vi "location calculator.vi"() -> ()   [LabVIEW 2015]
panel:
  out "1-D Array of Real":dbl[](array[numeric])
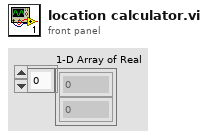
[diagram p1: front panel]
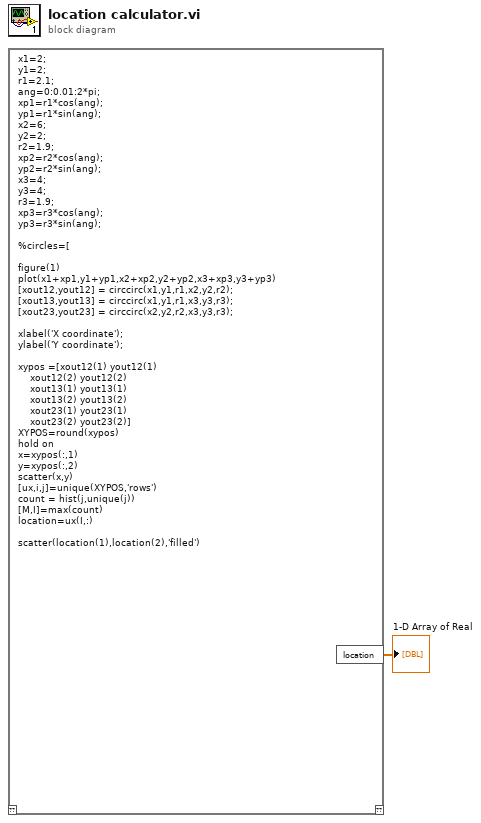
[diagram p0: block diagram]
diagram:
  n1 = script code="x1=2;\ny1=2;\nr1=2.1;\nang=0:0.01:2*pi;\nxp1=r1*cos(ang);\nyp1=r1*sin(ang);\nx2=6;\ny2=2;\nr2=1.9;\nxp2=r2*cos(ang);\nyp2=r2*sin(ang);\nx3=4;\ny3=4;\nr3=1.9;\nxp3=r3*cos(ang);\nyp3=r3*sin(ang);\n\n%circles=[\n\nfigure(1)\nplot(x1+xp1,y1+yp1,x2+xp2,y2+yp2,x3+xp3,y3+yp3)\n[xout12,yout12] = circcirc(x1,y1,r1,x2,y2,r2);\n[xout13,yout13] = circcirc(x1,y1,r1,x3,y3,r3);\n[xout23,yout23] = circcirc(x2,y2,r2,x3,y3,r3);\n\nxlabel('X coordinate');\nylabel('Y coordinate');\n\nxypos =[xout12(1) yout12(1)\n    xout12(2) yout12(2)\n    xout13(1) yout13(1)\n    xout13(2) yout13(2)\n    xout23(1) yout23(1)\n    xout23(2) yout23(2)]\nXYPOS=round(xypos)\nhold on\nx=xypos(:,1)\ny=xypos(:,2)\nscatter(x,y)\n[ux,i,j]=unique(XYPOS,'rows')\ncount = hist(j,unique(j))\n[M,I]=max(count)\nlocation=ux(I,:)\n\nscatter(location(1),location(2),'filled')"() -> ("location"=→"1-D Array of Real":dbl[])  [unwired: 1 in, 1 out]
